vi "Send CTRL Notification.vi"(8 "error in (no error)":errorcluster, 10 "Control Data":T1, 11 "CTRL Data Notifier in":refnum<notifier>) -> (0 "error out":errorcluster, 3 "CTRL Data Notifier out":refnum<notifier>)   [LabVIEW 2014, in "WINFAS 2 Data Queue.lvlib"]
uses:
  WINFAS 2 Data Queue.lvlib
  Control Data Cluster.ctl
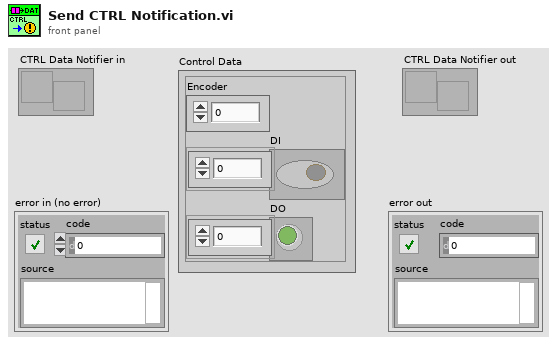
[diagram p1: front panel]
types:
  T1 = typedef "WINFAS 2 Data Queue.lvlib/Control Data Cluster.ctl" = cluster{"Encoder":sgl, "DI":bool[], "DO":bool[]}
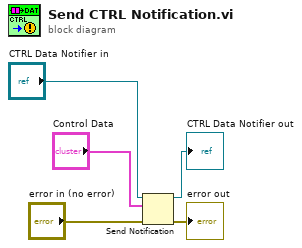
[diagram p0: block diagram]
diagram:
  n1 = Send Notification(notification="Control Data", notifier="CTRL Data Notifier in", error in (no error)="error in (no error)") -> (notifier out=→"CTRL Data Notifier out":refnum<notifier>, error out=→"error out":errorcluster)
